vi "Add.vi"(8 "error in (no error)":errorcluster, 10 "Equipment":refnum<class "Equipment.lvclass">, 11 "reference in":refnum<class "Rig.lvclass">) -> (0 "error out":errorcluster, 3 "reference in":refnum<class "Rig.lvclass">)   [LabVIEW 2020, in "Rig.lvclass"]
uses:
  Rig.lvclass
  Equipment_class/Equipment.lvclass
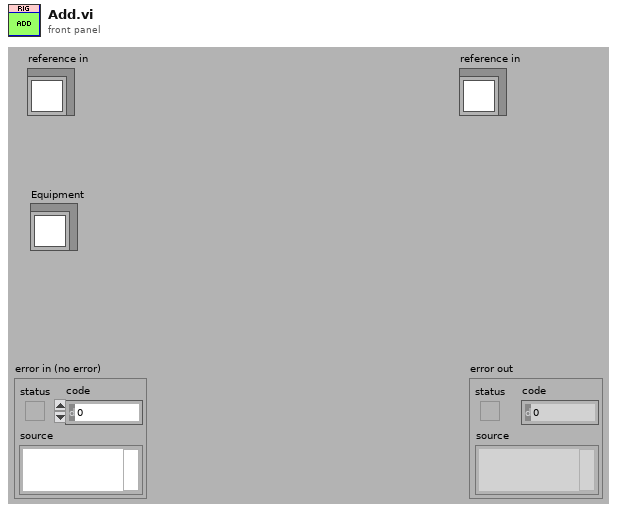
[diagram p1: front panel]
types:
  T1 = typedef "Rig.lvclass/ObjectAttributes.ctl" = cluster{"Children":refnum<class "Equipment.lvclass">[]}
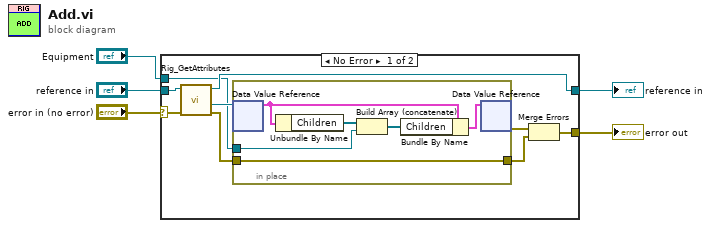
[diagram p0: block diagram]
diagram:
  n1 = case shown="No Error" "error in (no error)" {
    selector: "error in (no error)" -> [w13 w22]
    tunnel: [w11 w22] -> w4
    tunnel: [w10 w21] -> w2
    tunnel: "reference in" -> [w14 w21]
    tunnel: "Equipment" -> [w6 _]
    frame No Error {
      n2 = call "Rig_GetAttributes.vi"("error in (no error)"=w13, "reference in"=w14) -> ("error out"=w8:errorcluster, "DataRef"=w9:refnum<data-value>, "reference out"=w10:refnum<class "Rig.lvclass">)  [unwired: 6 in, 1 out]
      n3 = in-place {
        in-place-border: w8 -> [w19]
        in-place-border: [w19] -> w7
        in-place-border: w6 -> [w16]
        n4 = in-place-dvr #1(w9) -> (w18:T1)  [unwired: 1 out]
        n5 = Unbundle By Name(w18) -> ("Children"=w17:refnum<class "Equipment.lvclass">[])
        n6 = Build Array (concatenate)(w17, w16) -> (w15:refnum<class "Equipment.lvclass">[])
        n7 = Bundle By Name(cluster=w18, "Children"=w15) -> (w20:T1)
        n8 = in-place-dvr #1(w20) -> (w12:errorcluster)  [unwired: 1 out]
      }
      n9 = Merge Errors(w12, w7) -> (w11:errorcluster)
    }
    frame Error {
    }
  }
  "error out" <- w4
  "reference in" <- w2
